vi "Convert_FaultTable.vi"(0 "ERD Data Out":T2[](array[typedef]) {"ERD Number" format="%.0x"}, 11 "Error In":errorcluster) -> (3 "Fault Entry 0":T1, 4 "Fault Entry 1":T1, 5 "I0Fault ID":string, 6 "Fault Entry 2":T1, 7 "I0Fault Status":string, 8 "Fault Entry 3":T1, 10 "Fault Entry 4":T1, 15 "Error Out":errorcluster)   [LabVIEW 2016, in "2015 VA Washer.lvlib"]
uses:
  Projects/2015 VA Washer.lvlib
  Common/LabVIEW GEA2 Toolkit/LabVIEW_GEA2_Toolkit.lvlibp/type defs/ERD Read Data Out.ctl
  type defs/Fault_Table_Information.ctl
  Common/LabVIEW GEA2 Toolkit/LabVIEW_GEA2_Toolkit.lvlibp
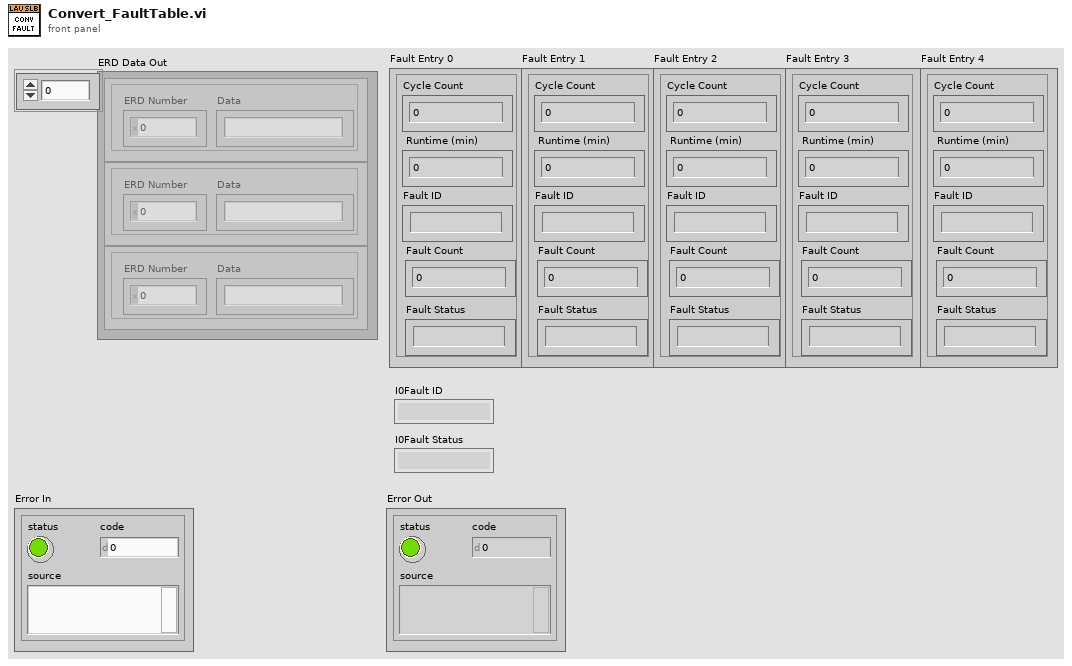
[diagram p1: front panel]
types:
  T1 = typedef "2015 VA Washer.lvlib/Fault_Table_Information.ctl" = cluster{"Cycle Count":u32, " Runtime (min) ":u32, "Fault ID":string, "Fault Count":u32, "Fault Status":string}
  T2 = typedef "LabVIEW_GEA2_Toolkit.lvlibp/ERD Read Data Out.ctl" = cluster{"ERD Number":u16, "Data":string}
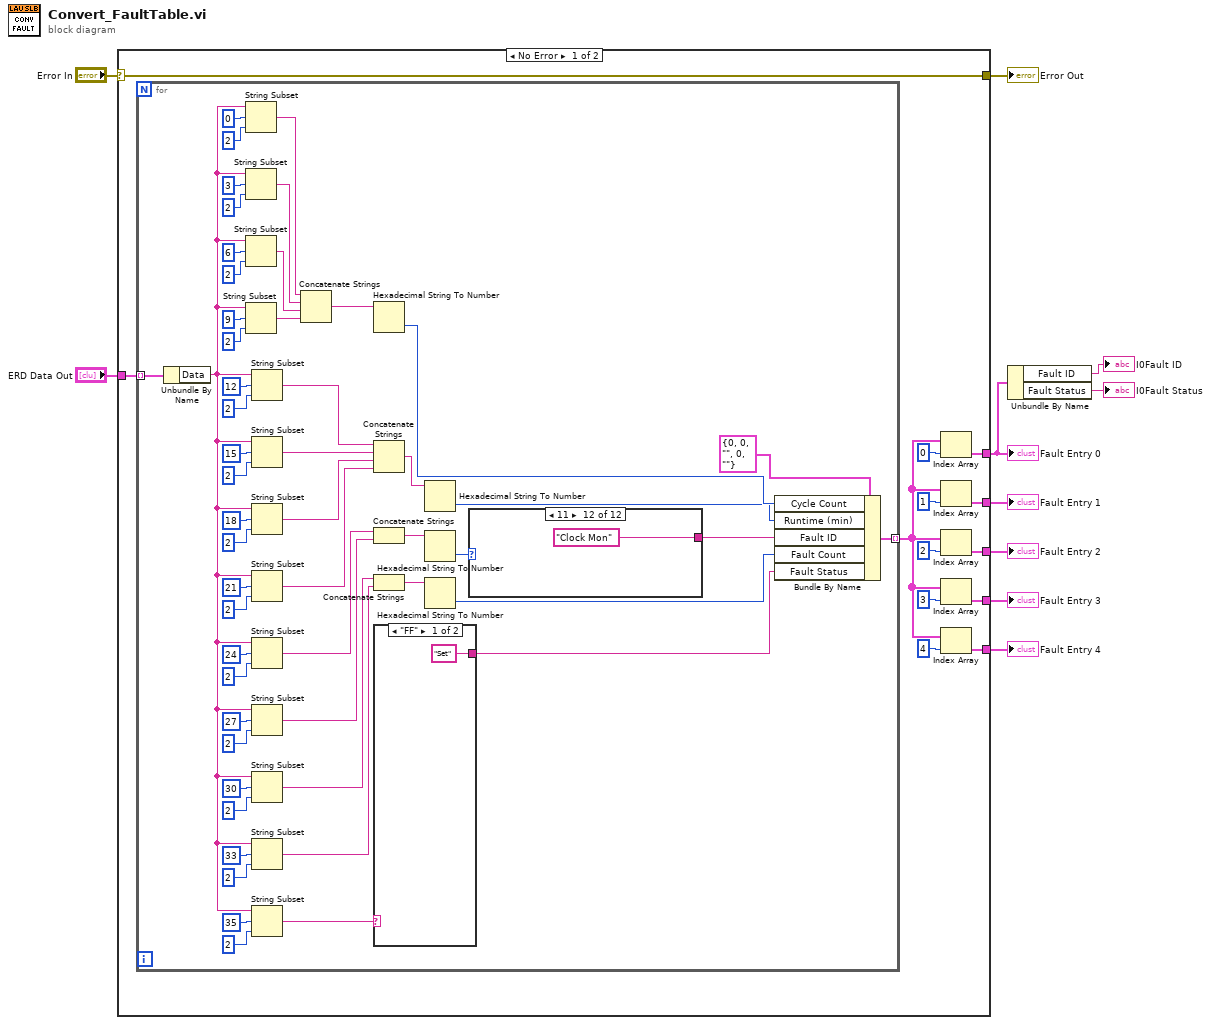
[diagram p0: block diagram]
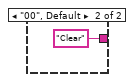
[diagram p2: hidden frame]
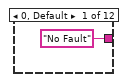
[diagram p3: hidden frame]
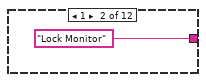
[diagram p4: hidden frame]
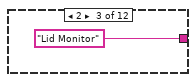
[diagram p5: hidden frame]
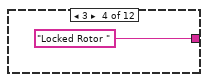
[diagram p6: hidden frame]
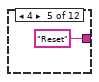
[diagram p7: hidden frame]
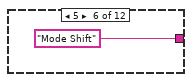
[diagram p8: hidden frame]
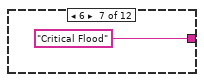
[diagram p9: hidden frame]
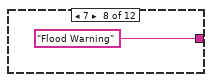
[diagram p10: hidden frame]
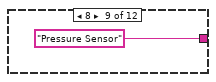
[diagram p11: hidden frame]
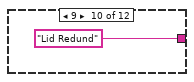
[diagram p12: hidden frame]
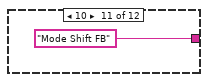
[diagram p13: hidden frame]
diagram:
  n1 = case shown="No Error" "Error In" {
    selector: "Error In" -> [w22 w91]
    tunnel: [w22 w91] -> w9
    tunnel: "ERD Data Out" -> [w23 _]
    tunnel: [w15 _] -> w3
    tunnel: [w14 _] -> w7
    tunnel: [w13 _] -> w6
    tunnel: [w12 _] -> w5
    tunnel: [w11 _] -> w4
    frame No Error {
      n2 = for {
        tunnel: w23 -> [w37] mode=indexing
        tunnel: [w25] -> w16 mode=indexing
        n3 = Unbundle By Name(w37) -> ("Data"=w32:string)
        n4 = String Subset(string=w32, offset (0)=0, length (rest)=2 ("length (rest)")) -> (substring=w72:string)
        n5 = String Subset(string=w32, offset (0)=3, length (rest)=2 ("length (rest)")) -> (substring=w71:string)
        n6 = String Subset(string=w32, offset (0)=6, length (rest)=2 ("length (rest)")) -> (substring=w70:string)
        n7 = String Subset(string=w32, offset (0)=9, length (rest)=2 ("length (rest)")) -> (substring=w69:string)
        n8 = String Subset(string=w32, offset (0)=12, length (rest)=2 ("length (rest)")) -> (substring=w62:string)
        n9 = String Subset(string=w32, offset (0)=15, length (rest)=2 ("length (rest)")) -> (substring=w63:string)
        n10 = String Subset(string=w32, offset (0)=18, length (rest)=2 ("length (rest)")) -> (substring=w64:string)
        n11 = String Subset(string=w32, offset (0)=21, length (rest)=2 ("length (rest)")) -> (substring=w65:string)
        n12 = String Subset(string=w32, offset (0)=24, length (rest)=2 ("length (rest)")) -> (substring=w55:string)
        n13 = String Subset(string=w32, offset (0)=27, length (rest)=2 ("length (rest)")) -> (substring=w54:string)
        n14 = String Subset(string=w32, offset (0)=30, length (rest)=2 ("length (rest)")) -> (substring=w30:string)
        n15 = String Subset(string=w32, offset (0)=33, length (rest)=2 ("length (rest)")) -> (substring=w29:string)
        n16 = String Subset(string=w32, offset (0)=35, length (rest)=2 ("length (rest)")) -> (substring=w24:string)
        n17 = Concatenate Strings(w72, w71, w70, w69) -> (w68:string)
        n18 = Hexadecimal String To Number(string=w68) -> (number=w67:u32)  [unwired: 2 in, 1 out]
        n19 = Concatenate Strings(w62, w63, w64, w65) -> (w66:string)
        n20 = Concatenate Strings(w55, w54) -> (w53:string)
        n21 = Concatenate Strings(w30, w29) -> (w31:string)
        n22 = case shown="\"FF\"" w24 {
          tunnel: ["Set" "Clear"] -> w27
          frame "FF" {
          }
          frame "00", Default {
          }
        }
        n23 = Hexadecimal String To Number(string=w66) -> (number=w50:u32)  [unwired: 2 in, 1 out]
        n24 = Hexadecimal String To Number(string=w53) -> (number=w52:u32)  [unwired: 2 in, 1 out]
        n25 = Hexadecimal String To Number(string=w31) -> (number=w26:u32)  [unwired: 2 in, 1 out]
        n26 = case shown="11" w52 {
          tunnel: ["No Fault" "Lock Monitor" "Lid Monitor" "Locked Rotor " "Reset" "Mode Shift" "Critical Flood" "Flood Warning" "Pressure Sensor" "Lid Redund" "Mode Shift FB" "Clock Mon"] -> w28
          frame 0, Default {
          }
          frame 1 {
          }
          frame 2 {
          }
          frame 3 {
          }
          frame 4 {
          }
          frame 5 {
          }
          frame 6 {
          }
          frame 7 {
          }
          frame 8 {
          }
          frame 9 {
          }
          frame 10 {
          }
          frame 11 {
          }
        }
        n27 = Bundle By Name(cluster=T1 {"Cycle Count"=0, " Runtime (min) "=0, "Fault ID"="", "Fault Count"=0, "Fault Status"=""} ("Fault Entry 2"), "Cycle Count"=w67, "Runtime (min)"=w50, "Fault ID"=w28, "Fault Count"=w26, "Fault Status"=w27) -> (w25:T1)
      }
      n28 = Index Array(array=w16, index=0) -> (element=w15:T1)
      n29 = Index Array(array=w16, index=1) -> (element=w14:T1)
      n30 = Index Array(array=w16, index=2) -> (element=w13:T1)
      n31 = Index Array(array=w16, index=3) -> (element=w12:T1)
      n32 = Index Array(array=w16, index=4) -> (element=w11:T1)
    }
    frame Error {
    }
  }
  "Error Out" <- w9
  "Fault Entry 1" <- w7
  "Fault Entry 2" <- w6
  "Fault Entry 3" <- w5
  "Fault Entry 4" <- w4
  "Fault Entry 0" <- w3
  n33 = Unbundle By Name(w3) -> ("Fault ID"=→"I0Fault ID":string, "Fault Status"=→"I0Fault Status":string)
